vi "Card Output Q.vi"(7 "Action":enum16{"Initial", "Write", "Read", "Release"}(ring)=enum."Release", 8 "error In":errorcluster, 10 "CardIndex":i32, 11 "OutputQIn":refnum<queue>) -> (0 "error Out":errorcluster, 3 "Output Q Out":refnum<queue>)   [LabVIEW 2019, in "IOCard.lvclass"]
uses:
  IOCard.lvclass
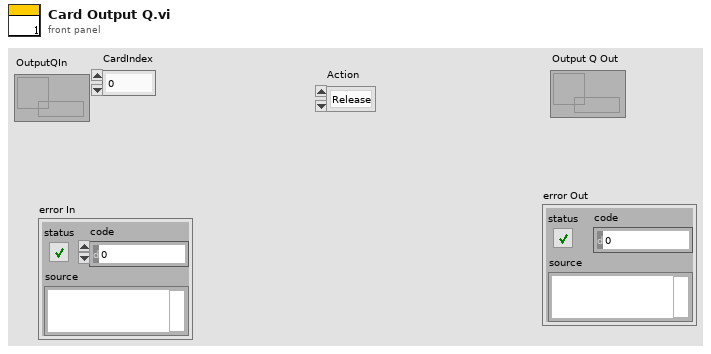
[diagram p1: front panel]
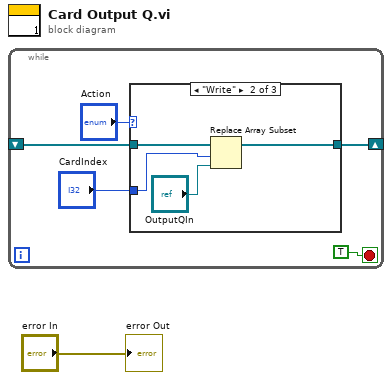
[diagram p0: block diagram]
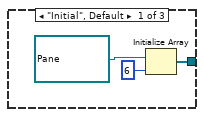
[diagram p2: hidden frame]
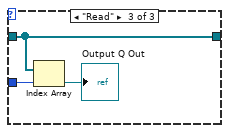
[diagram p3: hidden frame]
diagram:
  n1 = while {
    shift-right: [w4] -> _
    shift-left: _ -> [w3]
    stop <- TRUE stop-if-true
    n2 = case shown="\"Write\"" "Action" {
      tunnel: [w7 w12 w15] -> w4
      tunnel: w3 -> [_ w13 w15]
      tunnel: "CardIndex" -> [_ w10 w16]
      frame "Initial", Default {
        n3 = Initialize Array(refnum<queue> refnum ("OutPut QIn"), 6 ("dimension size")) -> (w7:refnum<queue>[])
      }
      frame "Write" {
        n4 = Replace Array Subset(array=w13, new element="OutputQIn", index=w10) -> (w12:refnum<queue>[])
      }
      frame "Read" {
        n5 = Index Array(array=w15, index=w16) -> (element=→"Output Q Out":refnum<queue>)
      }
    }
  }
  "error Out" <- "error In"
